vi "AdjustFrontPanelPosition.vi"(0 "Up":bool, 1 "Left":bool, 2 "Right":bool, 3 "Down":bool, 4 "Front Panel Reference":refnum<vi>) -> (5 "Top Position":i32, 6 "Left Position":i32)   [LabVIEW 2018]
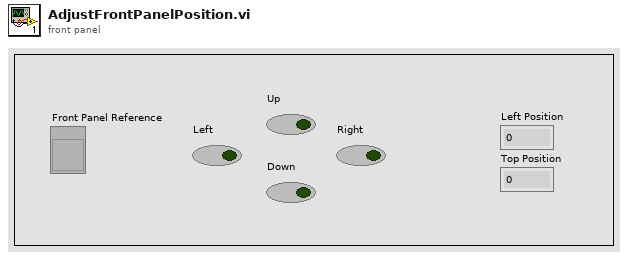
[diagram p1: front panel]
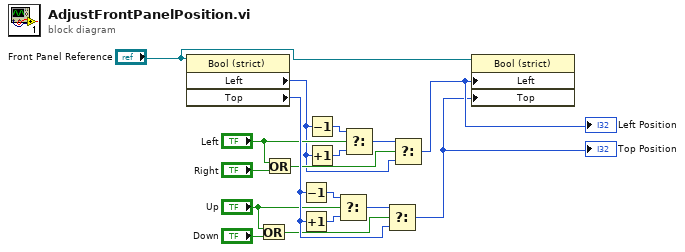
[diagram p0: block diagram]
diagram:
  n1 = property class="Bool (strict)"(reference="Front Panel Reference") -> ("Left"=w4:i32, "Top"=w14:i32)  [unwired: 1 in, 2 out]
  n2 = Or(x="Up", y="Down") -> (x .or. y?=w11:bool)
  n3 = Or(x="Left", y="Right") -> (x .or. y?=w5:bool)
  n4 = Decrement(x=w14) -> (x-1=w17:i32)
  n5 = Increment(x=w14) -> (x+1=w16:i32)
  n6 = Decrement(x=w4) -> (x-1=w10:i32)
  n7 = Increment(x=w4) -> (x+1=w9:i32)
  n8 = Select(t=w17, s="Up", f=w16) -> (s? t:f=w15:i32)
  n9 = Select(t=w10, s="Left", f=w9) -> (s? t:f=w8:i32)
  n10 = Select(t=w15, s=w11, f=w14) -> (s? t:f=w1:i32)
  "Top Position" <- w1
  n11 = Select(t=w8, s=w5, f=w4) -> (s? t:f=w3:i32)
  "Left Position" <- w3
  n12 = property class="Bool (strict)"(reference="Front Panel Reference", "Left"=w3, "Top"=w1) -> ()  [unwired: 1 in, 2 out]
